vi "Example Get Device Information.vi"() -> ()   [LabVIEW 2021]
doc: "This VI example shows how to get the information of the instrument U1282A."
uses:
  Keysight U1282A.lvlib
panel:
  in  "VISA resource name":refnum<visa-resource-name>="Keysight_U1282A"
  out "Firmware Revision":string
  out "Serial Number":string
  out "Manufacturer":string
  out "Model Number":string
  # "This VI example shows how to obtain the information of the instrument U1282A."
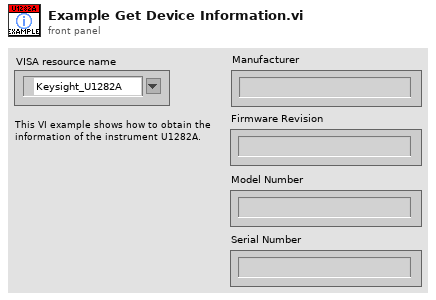
[diagram p1: front panel]
types:
  T1 = cluster{"Baud Rate":enum16{"1200", "2400", "4800", "9600", "19200", "38400", "57600", "115200"}, "Timeout":u32, "Stop Bits":u16, "Flow Control":enum16{"None", "XON / XOFF", "RTS / CTS", "DTR / DSR"}, "Parity":u16}
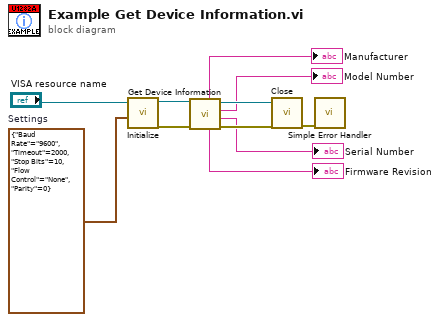
[diagram p0: block diagram]
diagram:
  w7 = T1 {"Baud Rate"=enum."9600", "Timeout"=2000, "Stop Bits"=10, "Flow Control"=enum."None", "Parity"=0}  # Settings
  n1 = call "Initialize.vi"("Settings"=w7, "VISA resource name"="VISA resource name") -> ("error out"=w10:errorcluster, "VISA resource name out"=w11:refnum<visa-resource-name>)  [unwired: 8 in]
  n2 = call "Get Device Information.vi"("error in"=w10, "VISA resource name in"=w11) -> ("error out"=w9:errorcluster, "Serial Number"=→"Serial Number":string, "Model Number"=→"Model Number":string, "VISA resource name out"=w8:refnum<visa-resource-name>, "Firmware Revision"=→"Firmware Revision":string, "Manufacturer"=→"Manufacturer":string)  [unwired: 4 in]
  n3 = call "Close.vi"("error in"=w9, "VISA resource name"=w8) -> ("error out"=w1:errorcluster)  [unwired: 9 in]
  n4 = call <vilib>:"Simple Error Handler.vi"("error in (no error)"=w1) -> ()  [unwired: 4 in, 5 out]
